vi "Update Live Data.vi"(8 "error in (no error)":errorcluster caption="错误输入（无错误）", 10 "new waveform array":waveform(dbl)[](array[waveform]) caption="新波形数组", 11 "original waveform array":waveform(dbl)[](array[waveform]) caption="原波形数组") -> (0 "error out":errorcluster caption="错误输出", 2 "min duration":dbl caption="最小时长", 3 "updated wavefrom array":waveform(dbl)[](array[waveform]) caption="更新后波形数组")   [LabVIEW 2015]
uses:
  Globals/Global - Monitoring Variables.vi
  <vilib>/Waveform/WDTOps.llb/WDT Index Channel DBL.vi
  <vilib>/Waveform/WDTOps.llb/WDT Append Waveforms DBL.vi
  <vilib>/Waveform/WDTOps.llb/WDT Waveform Duration DBL.vi
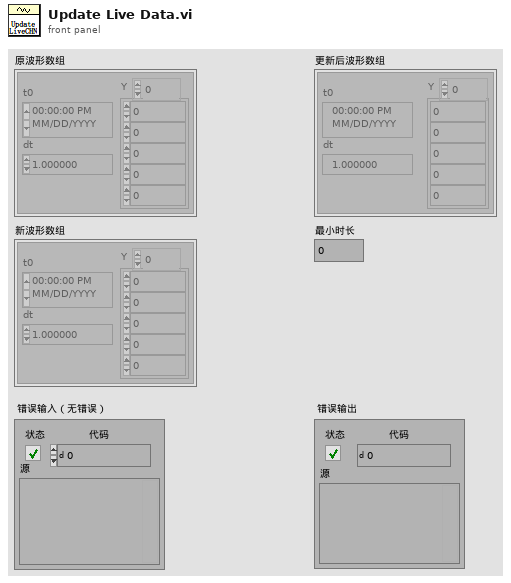
[diagram p1: front panel]
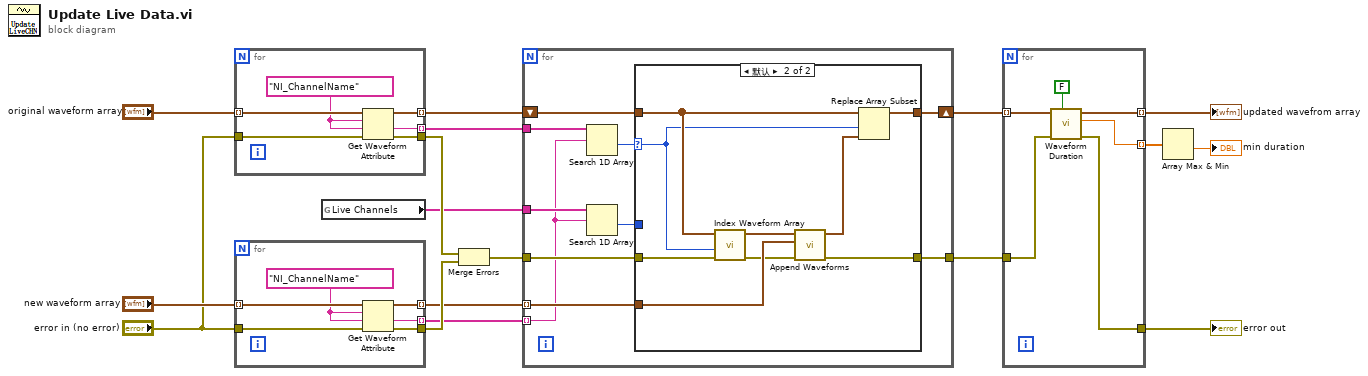
[diagram p0: block diagram]
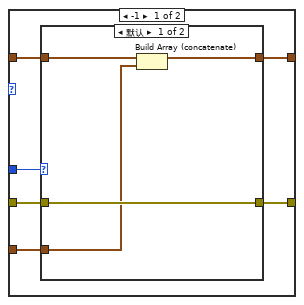
[diagram p2: hidden frame]
diagram:
  n1 = for {
    tunnel: "original waveform array" -> [w23] mode=indexing
    tunnel: "error in (no error)" -> [w22]
    tunnel: [w20] -> w17 mode=indexing
    tunnel: [w19] -> w16 mode=indexing
    tunnel: [w18] -> w14
    w21 = "NI_ChannelName" ("名称")
    n2 = Get Waveform Attribute(4:w22, 5:w21, 6:w21, 7:w23) -> (0:w18:errorcluster, 1:w20:string, 3:w19:waveform(dbl))  [unwired: 1 out]
  }
  n3 = for {
    tunnel: "new waveform array" -> [w29] mode=indexing
    tunnel: "error in (no error)" -> [w28]
    tunnel: [w26] -> w13 mode=indexing
    tunnel: [w25] -> w12 mode=indexing
    tunnel: [w24] -> w15
    w27 = "NI_ChannelName" ("名称")
    n4 = Get Waveform Attribute(4:w28, 5:w27, 6:w27, 7:w29) -> (0:w24:errorcluster, 1:w26:string, 3:w25:waveform(dbl))  [unwired: 1 out]
  }
  n5 = global read "Global - Monitoring Variables.vi" "Live Channels"() -> (w1:string[])
  n6 = Merge Errors(w14, w15) -> (w11:errorcluster)
  n7 = for {
    tunnel: w17 -> [w33]
    tunnel: w13 -> [w32] mode=indexing
    tunnel: w12 -> [w38] mode=indexing
    shift-right: [w36] -> w10
    shift-left: w16 -> [w37]
    tunnel: w11 -> [w39]
    tunnel: [w35] -> w9
    tunnel: w1 -> [w34]
    n8 = Search 1D Array(1D array=w33, element=w32) -> (index of element=w31:i32)  [unwired: 1 in]
    n9 = Search 1D Array(1D array=w34, element=w32) -> (index of element=w30:i32)  [unwired: 1 in]
    n10 = case shown="默认" w31 {
      selector: w31 -> [_ w52]
      tunnel: w37 -> [w43 w56]
      tunnel: w39 -> [w41 w60]
      tunnel: w38 -> [w40 w59]
      tunnel: [w44 w58] -> w36
      tunnel: [w42 w57] -> w35
      tunnel: w30 -> [w45 _]
      frame -1 {
        n11 = case shown="默认" w45 {
          tunnel: [w47 w51] -> w44
          tunnel: w43 -> [w48 w51]
          tunnel: [w49 w50] -> w42
          tunnel: w41 -> [w49 w50]
          tunnel: w40 -> [w46 _]
          frame Default {
            n12 = Build Array (concatenate)(w48, w46) -> (w47:waveform(dbl)[])
          }
          frame -1 {
          }
        }
      }
      frame Default {
        n13 = call-poly <vilib>:"Index Waveform Array.vi"("error in (no error)"=w60, "index"=w52, "waveform array"=w56) -> ("error out"=w54:errorcluster, "waveform"=w55:waveform(dbl))  [unwired: 7 in]
        n14 = call-poly <vilib>:"Append Waveforms.vi"("error in (no error)"=w54, "waveform B"=w59, "waveform A"=w55) -> ("error out"=w57:errorcluster, "waveform out"=w53:waveform(dbl))  [unwired: 7 in]
        n15 = Replace Array Subset(array=w56, new element=w53, index=w52) -> (w58:waveform(dbl)[])
      }
    }
  }
  n16 = for {
    tunnel: w10 -> [w66] mode=indexing
    tunnel: [w65] -> w4 mode=indexing
    tunnel: w9 -> [w64]
    tunnel: [w63] -> w2
    tunnel: [w62] -> w8 mode=indexing
    n17 = call-poly <vilib>:"Waveform Duration.vi"("open interval? (T)"=FALSE, "error in (no error)"=w64, "waveform in"=w66) -> ("error out"=w63:errorcluster, "duration"=w62:dbl, "waveform out"=w65:waveform(dbl))  [unwired: 6 in]
  }
  "error out" <- w2
  "updated wavefrom array" <- w4
  n18 = Array Max & Min(array=w8) -> (min value=→"min duration":dbl)  [unwired: 3 out]
